vi "Window-controller response_v0.vi"() -> ()   [LabVIEW 2020]
panel:
  out "size(s)":i32
  out "Array":T1(array[cluster])
  in  "stop":bool
  out "Packet Data:":string
  out "Good Read":bool
  out "Timeout":bool
  out "Read Error":bool
  out "Pkt Len":i32
  out "Pkt uSec":i32
  out "Pkt Sec":i32
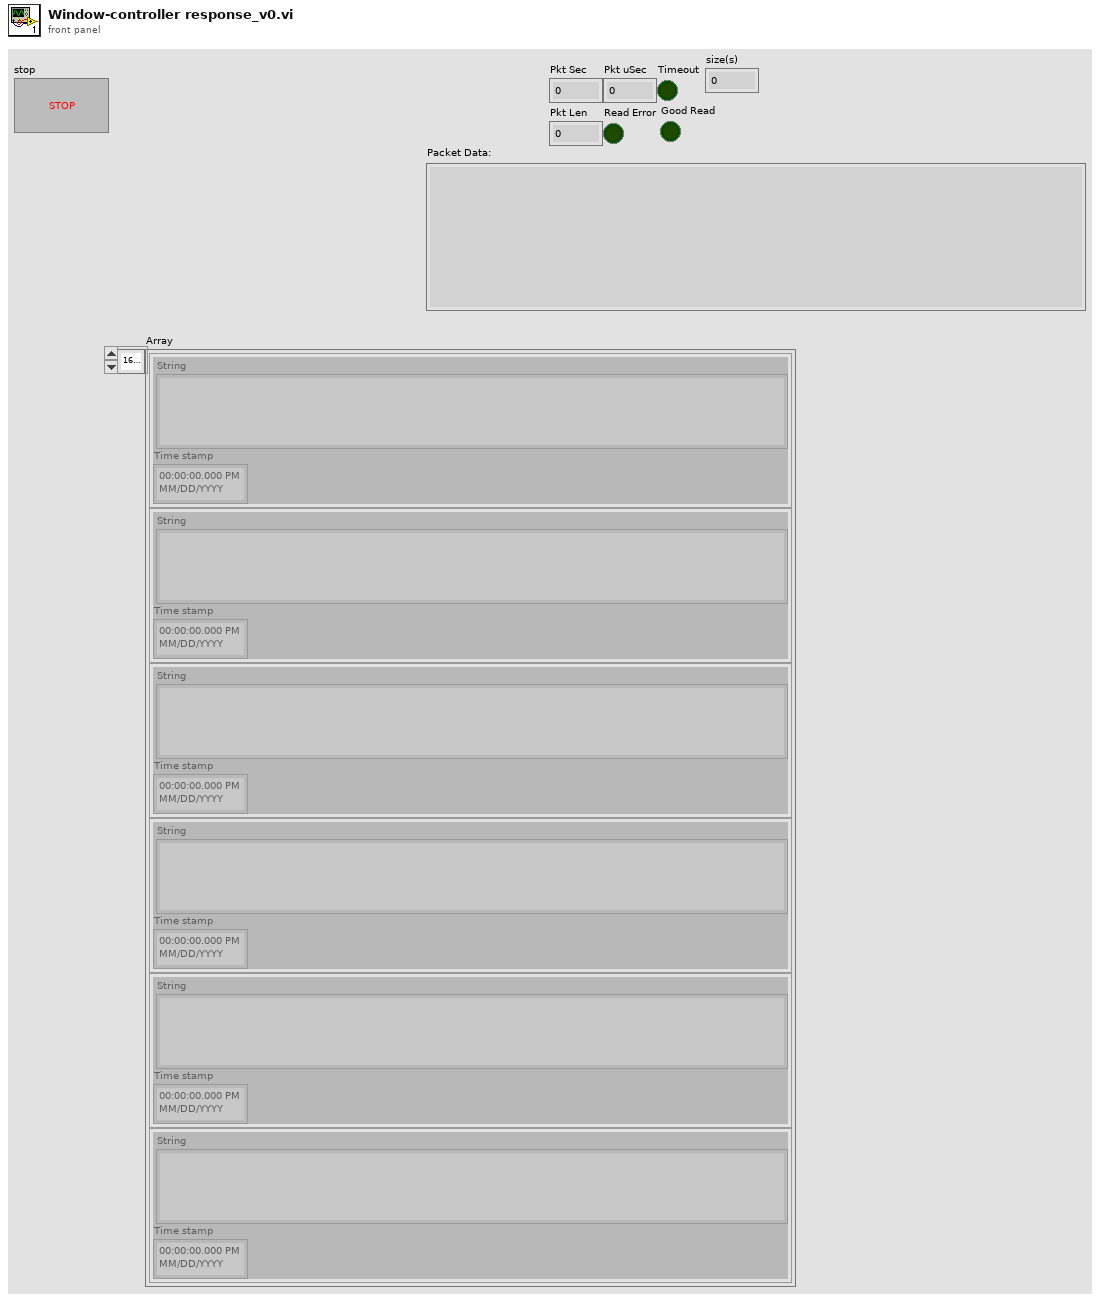
[diagram p1: front panel]
types:
  T1 = cluster{"String":string, "Time stamp":timestamp}[]
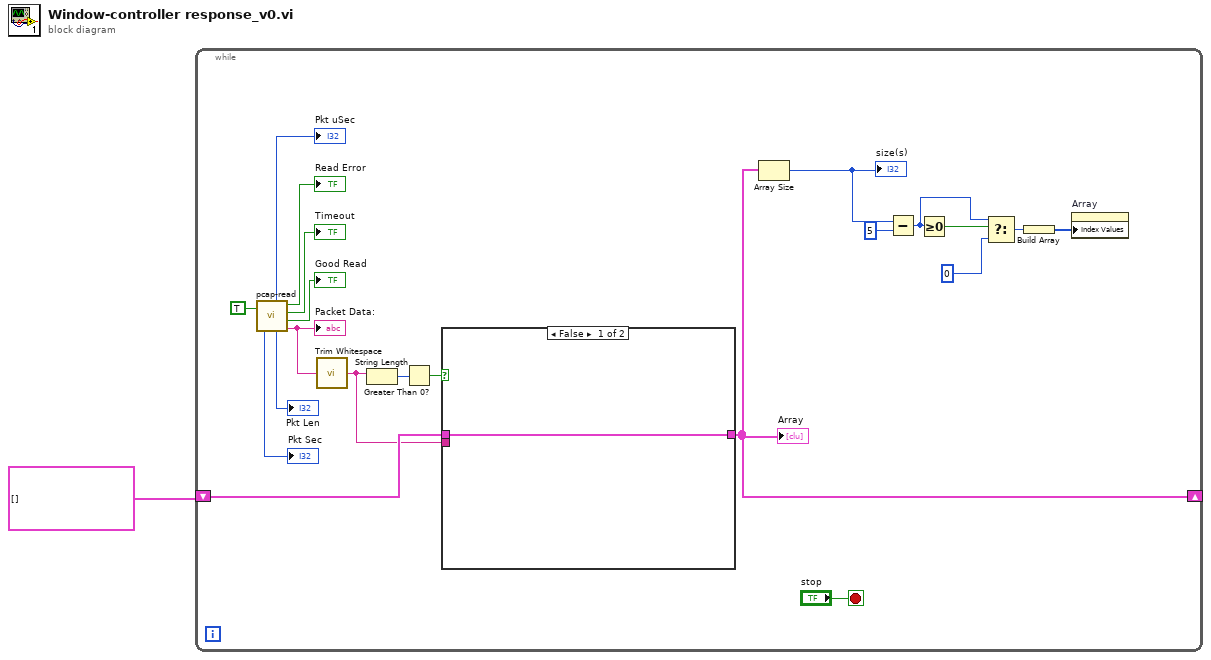
[diagram p0: block diagram]
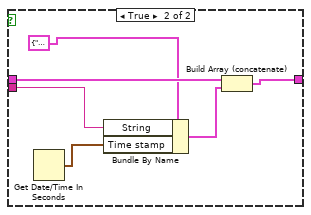
[diagram p2: hidden frame]
diagram:
  n1 = while {
    shift-right: [w9] -> _
    shift-left: T1 [] -> [w11]
    stop <- "stop" stop-if-true
    n2 = call "pcap-read.vi"("Opened"=TRUE) -> ("Pkt Sec"=→"Pkt Sec":i32, "Pkt uSec"=→"Pkt uSec":i32, "Pkt Len"=→"Pkt Len":i32, "Read Error"=→"Read Error":bool, "Timeout"=→"Timeout":bool, "Good Read"=→"Good Read":bool, "Packet Data:"=w14:string)
    "Packet Data:" <- w14
    n3 = call <vilib>:"Trim Whitespace.vi"("string"=w14) -> ("trimmed string"=w10:string)  [unwired: 1 in]
    n4 = String Length(string=w10) -> (length=w13:i32)
    n5 = Greater Than 0?(x=w13) -> (x > 0?=w12:bool)
    n6 = case shown="False" w12 {
      tunnel: w11 -> [w23 w29]
      tunnel: w10 -> [_ w28]
      tunnel: [w23 w24] -> w9
      frame False {
      }
      frame True {
        n7 = Get Date/Time In Seconds() -> (seconds since 1Jan1904=w26:timestamp)
        n8 = Bundle By Name(cluster=cluster{"String":string, "Time stamp":timestamp} {"String"="", "Time stamp"=timestamp(0 s since 1904-01-01)}, "String"=w28, "Time stamp"=w26) -> (w25:cluster{"String":string, "Time stamp":timestamp})
        n9 = Build Array (concatenate)(w29, w25) -> (w24:T1)
      }
    }
    "Array" <- w9
    n10 = Array Size(array=w9) -> (size(s)=w8:i32)
    "size(s)" <- w8
    n11 = Subtract(x=w8, y=5) -> (x-y=w4:i32)
    n12 = Greater Or Equal To 0?(x=w4) -> (x >= 0?=w6:bool)
    n13 = Select(t=w4, s=w6, f=0) -> (s? t:f=w3:i32)
    n14 = Build Array(w3) -> (w2:i32[])
    n15 = property on="Array" class="Arr (strict)"("Index Values"=w2) -> ()  [unwired: 2 in, 2 out]
  }
